vi "rsp_New Connection.vi"(4 "Show in Debugger?":bool=TRUE, 6 "Message Priority":T1=enum."Normal", 8 "error in":errorcluster, 10 "Data in":T2, 11 "gRPC Read in":refnum<class "gRPC Read.lvclass">) -> (0 "error out":errorcluster, 3 "dup gRPC Read out":refnum<class "gRPC Read.lvclass">)   [LabVIEW 2019, in "gRPC Server (template.proto).lvlib" / "gRPC Read.lvclass"]
doc: "This VI sends a <b>Public API Response</b> message to a registered MHL case of the Caller of the Worker that owns this VI.\n---\nA new connection has been established with a gRPC Client."
uses:
  gRPC Read.lvclass
  gRPC Read.lvclass/gRPC Read.ctl
  <vilib>/ErrorRing/Error Ring.xnode
  <vilib>/addons/_Workers/Library/Classes/Worker/Worker.lvclass
  <vilib>/Utility/error.llb/Error Cluster From Error Code.vi
  <vilib>/addons/_Workers/Library/Classes/Message/Priority.ctl
  <vilib>/addons/_Workers/Library/Classes/Message/Message.lvclass
  rsp_New Connection.ctl
  <vilib>/gRPC/LabVIEW gRPC Library/Shared/grpcId.ctl
  <vilib>/gRPC/LabVIEW gRPC Library/grpc-lvsupport-release.lvlib
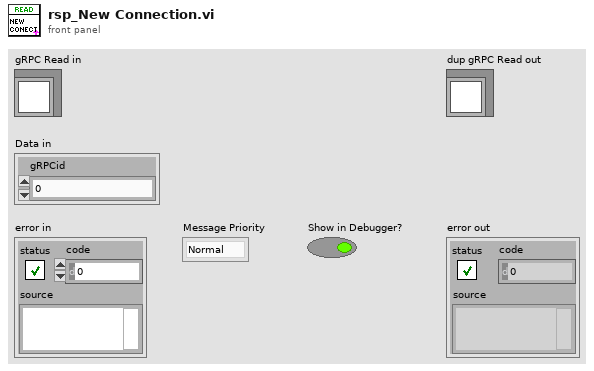
[diagram p1: front panel]
types:
  T1 = typedef "Workers.lvlib/Message.lvclass/Priority.ctl" = enum16{"Low", "Normal", "High"}
  T2 = typedef "gRPC Server (template.proto).lvlib/gRPC Read.lvclass/rsp_New Connection.ctl" = cluster{"gRPCid":T3}
  T3 = typedef "grpc-lvsupport-release.lvlib/grpcId.ctl" = u64
  T4 = typedef "Workers.lvlib/Case Label.ctl" = string
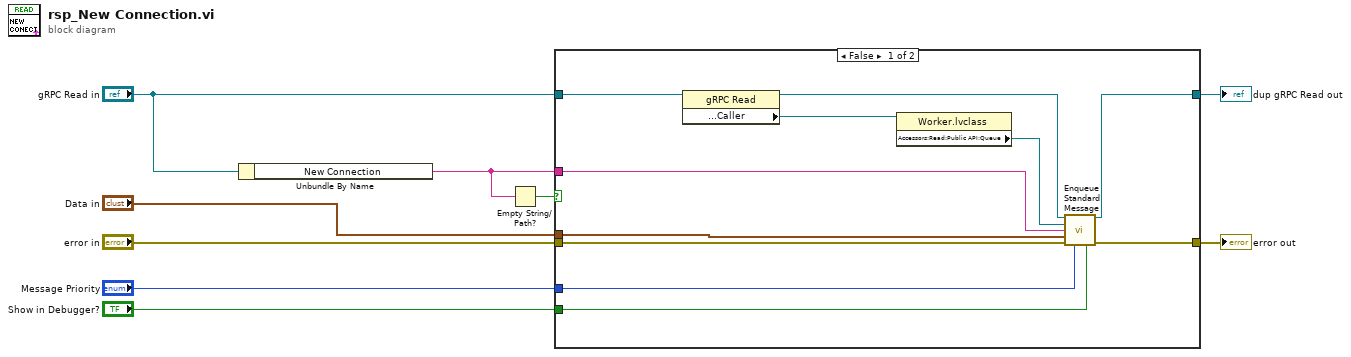
[diagram p0: block diagram]
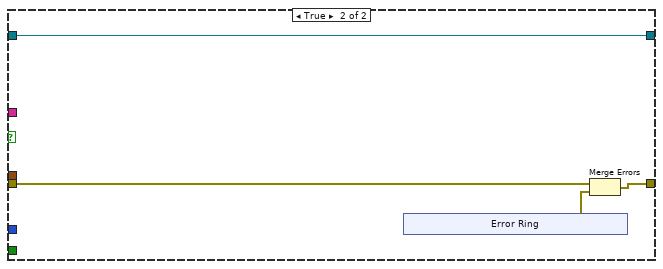
[diagram p2: hidden frame]
diagram:
  n1 = Unbundle By Name("gRPC Read in") -> ("New Connection"=w4:T4)
  n2 = Empty String/Path?(string/path=w4) -> (empty?=w5:bool)
  n3 = case shown="False" w5 {
    tunnel: "error in" -> [w20 w21]
    tunnel: [w19 w22] -> w8
    tunnel: "Data in" -> [w16 _]
    tunnel: [w18 w24] -> w6
    tunnel: "gRPC Read in" -> [w13 w24]
    tunnel: w4 -> [w17 _]
    tunnel: "Show in Debugger?" -> [w15 _]
    tunnel: "Message Priority" -> [w14 _]
    frame False {
      n4 = property class="gRPC Read"(reference=w13) -> (reference out=w12:refnum<class "gRPC Read.lvclass">, "Accessors:Read:Public API:Caller"=w10:refnum<class "Worker.lvclass">)  [unwired: 1 in, 1 out]
      n5 = property class="Worker.lvclass"(reference=w10) -> ("Accessors:Read:Public API:Queue"=w11:refnum<class "Message Queue.lvclass">)  [unwired: 1 in, 2 out]
      n6 = call-dynamic "Enqueue Standard Message.vi"("Worker"=w12, "Message Queue"=w11, "Case Label"=w17, "Data"=w16, "error in (no error)"=w20, "Priority (Normal)"=w14, "Send Message to Debugger? (T)"=w15) -> ("dup Worker out"=w18:refnum<class "gRPC Read.lvclass">, "error out"=w19:errorcluster)  [unwired: 7 in]
    }
    frame True {
      n7 = xnode "Error Ring"() -> ("error out"=w23:errorcluster)
      n8 = Merge Errors(w21, w23) -> (w22:errorcluster)
    }
  }
  "error out" <- w8
  "dup gRPC Read out" <- w6
